vi "AlliGator Get Local Fit & Residuals.vi"(6 "Fit Options":T1={"Show Fit Residuals"=TRUE, "Fit Model"=enum."1-Exponential", "Residual Type"=enum."Standard", "Max Decay Percentile"=0.0, "Min Decay Percentile"=0.0, "Show Full Decay"=TRUE, "Weights"=enum."Unweighted", "Fitting Method"=enum."Least Square", "Compute Parameter Uncertainties"=TRUE, "Periodic Boundaries"=TRUE, "Model Calculation"=enum."Simulation", "Period"=1.2500000000000001e-08, "Termination Criteria"={"Max Iterations"=0, "Max Function Calls"=0, "Max Time"=1000.0, "Function Tolerance"=1e-06, "Parameter Tolerance"=1e-06, "Gradient Tolerance"=0.0, "Min Lambda"=1e-06, "Max Lambda"=1e-06, "Initial Tick Count"=0}, "Offset Resolution"=1.2500000000000001e-08, "Use Local IRF"=TRUE, "Fitting Algorithm"=enum."Levenberg-Marquardt"} {"Offset Resolution" min=0.0; "Period" min=0.0; "Min Decay Percentile" min=0.0 max=1.0; "Max Decay Percentile" min=0.0 max=1.0}, 7 "Use Normalized IRF (T)":bool=TRUE, 8 "Error In":errorcluster, 9 "All Fit Parameters (w tau)":dbl[](array[numeric]), 10 "IRF":cluster{"X Array":dbl[], "Y Array":dbl[]}, 11 "Decay Plot":cluster{"X Array":dbl[], "Y Array":dbl[]}) -> (0 "Error Out":errorcluster, 1 "Fit Model":T2, 2 "Residual Plot":cluster{"X Array":dbl[], "Y Array":dbl[]}, 3 "Fit Plot":cluster{"X Array":dbl[], "Y Array":dbl[]})   [LabVIEW 2021, in "AlliGator Local Decay Window.lvlib"]
doc: "Gets the fit and residuals for the selected ROI."
uses:
  AlliGator Local Decay Window.lvlib
  Fits/Decay Convolution/Decay Model.ctl
  Fits/IRF(X)PSED/Decay Fit Options v2.ctl
  Fits/Residual Type.ctl
  Fits/IRF(X)PSED/Fit Weights Type.ctl
  Fits/Non-linear Fitting Method v2.ctl
  Fits/Fit Calculation Method.ctl
  Fits/Non-linear Fitting Algorithm.ctl
  AlliGator Settings List.ctl
  Variant/Variant to Data/Variant to Boolean.vi
  AlliGator Settings.lvlib
  Fits/Fits.lvlib
  Variant/Variant to Data/Variant to Data.lvlib
  AlliGator Decay Fit.lvlib
panel:
  # "see the AlliGator License on the block diagram (Ctrl+E or Window:Show Block Diagram)"
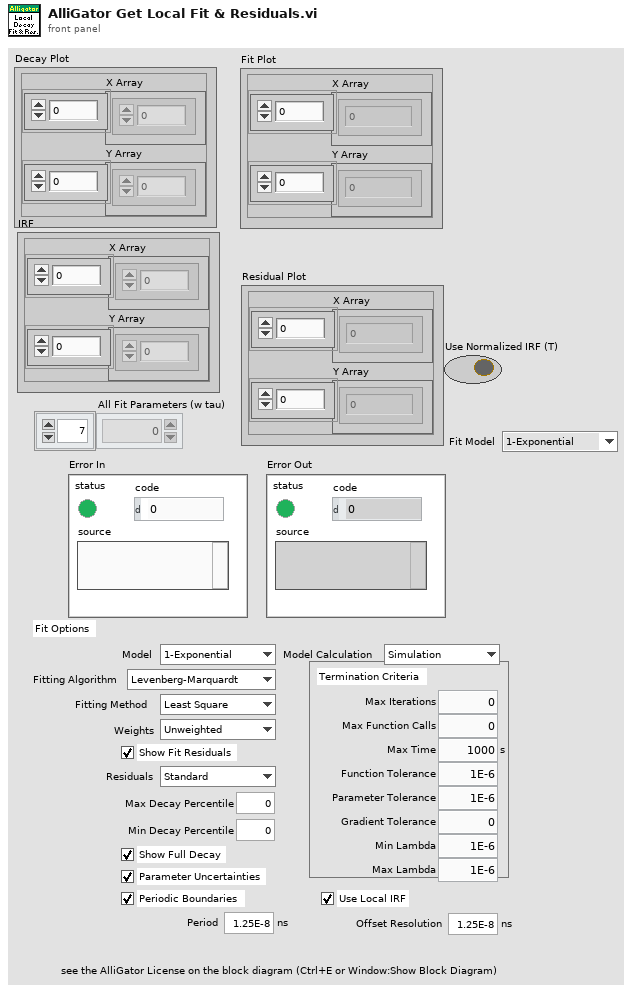
[diagram p1: front panel]
types:
  T1 = typedef "Fits.lvlib/Decay Fit Options v2.ctl" = cluster{"Show Fit Residuals":bool, "Fit Model":T2, "Residual Type":T3, "Max Decay Percentile":dbl, "Min Decay Percentile":dbl, "Show Full Decay":bool, "Weights":T4, "Fitting Method":T5, "Compute Parameter Uncertainties":bool, "Periodic Boundaries":bool, "Model Calculation":T6, "Period":dbl[unit], "Termination Criteria":cluster{"Max Iterations":i32, "Max Function Calls":i32, "Max Time":dbl[unit], "Function Tolerance":dbl, "Parameter Tolerance":dbl, "Gradient Tolerance":dbl, "Min Lambda":dbl, "Max Lambda":dbl, "Initial Tick Count":u32}, "Offset Resolution":dbl[unit], "Use Local IRF":bool, "Fitting Algorithm":T7}
  T2 = typedef "Fits.lvlib/Decay Model.ctl" = enum16{"1-Exponential", "2-Exponentials"}
  T3 = typedef "Fits.lvlib/Residual Type.ctl" = enum16{"Standard", "Normalized", "Reduced"}
  T4 = typedef "Fits.lvlib/Fit Weights Type.ctl" = enum16{"Unweighted", "1/Variance", "Best of All"}
  T5 = typedef "Fits.lvlib/Non-linear Fitting Method v2.ctl" = enum16{"Least Square", "Least Absolute Residual", "Bisquare", "MLE", "-", "Best of All"}
  T6 = typedef "Fits.lvlib/Fit Calculation Method.ctl" = enum16{"Simulation", "Convolution", "Integration"}
  T7 = typedef "Fits.lvlib/Non-linear Fitting Algorithm.ctl" = enum16{"Levenberg-Marquardt", "Trust-Region Dogleg"}
  T8 = typedef "AlliGator Settings.lvlib/AlliGator Settings List.ctl" = enum16{"GUI:Visible Settings Tab", "GUI:Last Run Version", "Source Image:Use Image Histogram for Contrast", "Source Image:Low Count Pixels Rejection Options", "Source Image:High Count Pixels Rejection Options", "Source Image:Use Image Brightness", "Source Image:Blend Overlay with Image Background", "Source Image:Use Fixed ROI Diameter", "Source Image:ROI Diameter", "Source Image:ROI Center Color", "Source Image:Peak Threshold", "Source Image:Intensity Threshold", "Source Image:Image Binning Options", "Source Image:Image Smoothing Options", "Source Image:Image Histogram Active", "Source Image:Invert Binary Mask", "Source Image:Hot Pixel Removal", "Source Image:Overlay Analyzed ROI Center", "Source Image:Auto-Adjust Contrast", "Source Image:Histogram Lower Percentile", "Source Image:Histogram Upper Percentile", "Source Image:Save Source Image", "Source Image:Scale Bar Options", "Source Image:Image Resolution (Pixel Size)", "Source Image:Flatfield Correction", "Source Image:Show Dead Left Columns Correction", "Source Image:Dead Left Columns Correction", "Source Image:Image Pre-Processing Operations Order", "Data Information:Gate Width", "Data Information:Nanotime Gate Separation", "Data Information:Macrotime Gate Separation", "Data Information:Gate Step", "Data Information:# Gates", "Data Information:Gate Image Exposure", "Data Information:Gate Image Integration", "Data Information:Gates to Skip", "Data Information:Gates to Keep", "Data Information:Define Gates to", "Data Information:Channel Name", "Data Information:Available Channel Names", "Data Information:Channel Arithmetic", "Data Information:Background File Subtraction", "Data Information:Background File", "Data Information:Background Scaling Factor", "Data Information:Background Pile-up Correction", "Data Information:Background Pixel Well Capacity", "Data Information:Laser Period", "Data Information:SYNC Period", "Data Information:Pile-up Correction", "Data Information:Pixel Well Capacity", "Data Information:Dataset Scaling Factor", "Fluorescence Decay_Decay Pre-Processing:Reverse Gates", "Fluorescence Decay_Decay Pre-Processing:Verbose Decay Pre-Processing", "Fluorescence Decay_Decay Pre-Processing:Use Decay Pre-Processing", "Fluorescence Decay_Decay Pre-Processing:Background Subtraction", "Fluorescence Decay_Decay Pre-Processing:Background Definition Range", "Fluorescence Decay_Decay Pre-Processing:Baseline Subtraction Method", "Fluorescence Decay_Decay Pre-Processing:Decay Pre-Processing Operations Order", "Fluorescence Decay_Decay Pre-Processing:Smoothing Parameter", "Fluorescence Decay_Decay Pre-Processing:Shift Decay", "Fluorescence Decay_Decay Pre-Processing:Decay Shift Parameters", "Fluorescence Decay_Decay Pre-Processing:Fold Decay", "Fluorescence Decay_Decay Pre-Processing:# Folds", "Fluorescence Decay_Decay Pre-Processing:1-Normalize Decay", "Fluorescence Decay_Decay Pre-Processing:[0-1]-Normalize Decay", "Fluorescence Decay_Decay Pre-Processing:Smoothen Decay", "Fluorescence Decay_Decay Pre-Processing:Extrapolate Decay", "Fluorescence Decay_Decay Pre-Processing:Use Periodicity", "Fluorescence Decay_Decay Pre-Processing:Use Cursors", "Fluorescence Decay_Decay Pre-Processing:Tail Fraction", "Fluorescence Decay_Decay Pre-Processing:Head Fraction", "Fluorescence Decay_Decay Pre-Processing:Additional Points", "Fluorescence Decay_Decay Pre-Processing:Straighten Decay", "Fluorescence Decay_Decay Pre-Processing:Constant Background", "Fluorescence Decay_Decay Pre-Processing:Pixel-Normalize Decay", "Fluorescence Decay_Advanced Analysis:Extract IRF instead of Decay", "Fluorescence Decay_Advanced Analysis:IRF Extraction Options", "Fluorescence Decay_Advanced Analysis:IRF Optimization Options", "Fluorescence Decay_Advanced Analysis:Square Pulse Options", "Fluorescence Decay_Advanced Analysis:IRF Order", "Fluorescence Decay_Advanced Analysis:IRF Time Constants", "Fluorescence Decay_Advanced Analysis:Wavelet Analysis Options", "Fluorescence Decay_Advanced Analysis:Average Lifetime Options", "Fluorescence Decay_Fit Options:Fit Options", "Fluorescence Decay_Fit Options:Use Legacy Fitting Approach", "Fluorescence Decay_Fit Options:Use Data Information Laser Period", "Fluorescence Decay_Fit Parameters:Displayed Fit Parameters", "Fluorescence Decay_Fit Parameters:Fit Parameter Constraints", "Fluorescence Decay_Fit Parameters:Export Tabulated Results", "Fluorescence Decay_Fit Parameters:MLE Baseline Offset Type", "Fluorescence Decay_Fit Parameters:MLE Baseline Offset", "Fluorescence Decay_Fit Parameters:Guess Parameter Names", "Fluorescence Decay_Fit Parameters:Guess Parameter Values", "Fluorescence Decay_Fit Parameters:Guess Parameters Options", "Fluorescence Decay_Styles:Show Last Decay Only", "Fluorescence Decay_Styles:Decay Graph Color Array", "Fluorescence Decay:Decay Graph Active", "Fluorescence Decay Statistics:Min Peak Value", "Fluorescence Decay Statistics:Reject Low Decay Peak Pixels", "Fluorescence Decay Statistics:Reject High Decay Peak Pixels", "Fluorescence Decay Statistics:Max Peak Value", "Time Traces:Use File Timestamp", "Time Traces:Time Step", "Time Traces:Use Intensity Correction File", "Time Traces:Intensity Correction File", "Phasor Plot:Phasor Plot Smoothing Options", "Phasor Plot:Phasor Plot Size", "Phasor Plot:Phasor Plot Graphics Options", "Phasor Plot:Cumulative Phasor Plot", "Phasor Plot:Use Phasor Brightness", "Phasor Plot:Blend Overlay with Phasor Background", "Phasor Plot:Save Phasor Plot", "Phasor Plot:Show References", "Phasor Plot:Phasor Ratio Decay Range", "Phasor Plot:Exponential Fading", "Phasor Plot:Phasor Ratio Reference Colors", "Phasor Plot:Reference Radius", "Phasor Plot:Show Color Map Vertices", "Phasor Plot:Phasor Plot Active", "Phasor Plot:Phasor Ratio Color Map Type", "Phasor Plot:Phasor Ratio Color Map", "Phasor Plot:Phasor Ratio Display Range", "Phasor Plot:Selected Image ROI(s)", "Phasor Plot:All Image ROIs", "Phasor Plot:Selected Phasor Plot ROI(s)", "Phasor Plot:All Phasor Plot ROIs", "Phasor Plot:Phasor Ratio Color-Coded Quantity", "Phasor Plot:Store Phasor Harmonics", "Phasor Plot:Draw Reference Segment", "Phasor Plot:User-Defined Quantity", "Phasor Graph:Phasor Frequency", "Phasor Graph:Phasor Ratio Type", "Phasor Graph:Pixel-level Phasor Computation", "Phasor Graph:Save Phasor Graph", "Phasor Graph:Phasor Graph Active", "Phasor Graph:Phasor SDV Options", "Phasor Calibration:Use Backup Calibration if needed", "Phasor Graph:Define Shortest Lifetime as", "Phasor Calibration:Backup Calibration Type", "Phasor Calibration:Calibration Type", "Phasor Calibration:Calibration Lifetime", "Phasor Calibration:Calibration Map Algorithm", "Single-Exponential Phasor Locus (SEPL):Gate Parameters", "Single-Exponential Phasor Locus (SEPL):User-defined Gate", "Single-Exponential Phasor Locus (SEPL):User-defined IRF", "Single-Exponential Phasor Locus (SEPL):Phasor Parameters", "Single-Exponential Phasor Locus (SEPL):Decay & IRF Parameters", "Single-Exponential Phasor Locus (SEPL):Display Parameters", "Lifetime Analysis:Decay Analysis Parameters", "Lifetime Analysis:Lifetime Map Active", "Plugins:Python Settings", "Miscellaneous:Verbose Mode", "Miscellaneous:Beep after Script", "Miscellaneous:Saved Image File Format", "Miscellaneous:Exported Gate Image Settings", "Miscellaneous:Include Loading in Timing", "Miscellaneous:Verbose Settings Mode", "Miscellaneous:Histogram Options", "Miscellaneous:Beep on Error", "Miscellaneous:# Logical Processors Used", "Miscellaneous:ROI Description Max Characters", "Miscellaneous:Verbose Error Mode", "Miscellaneous:Transparent Mask Color"}
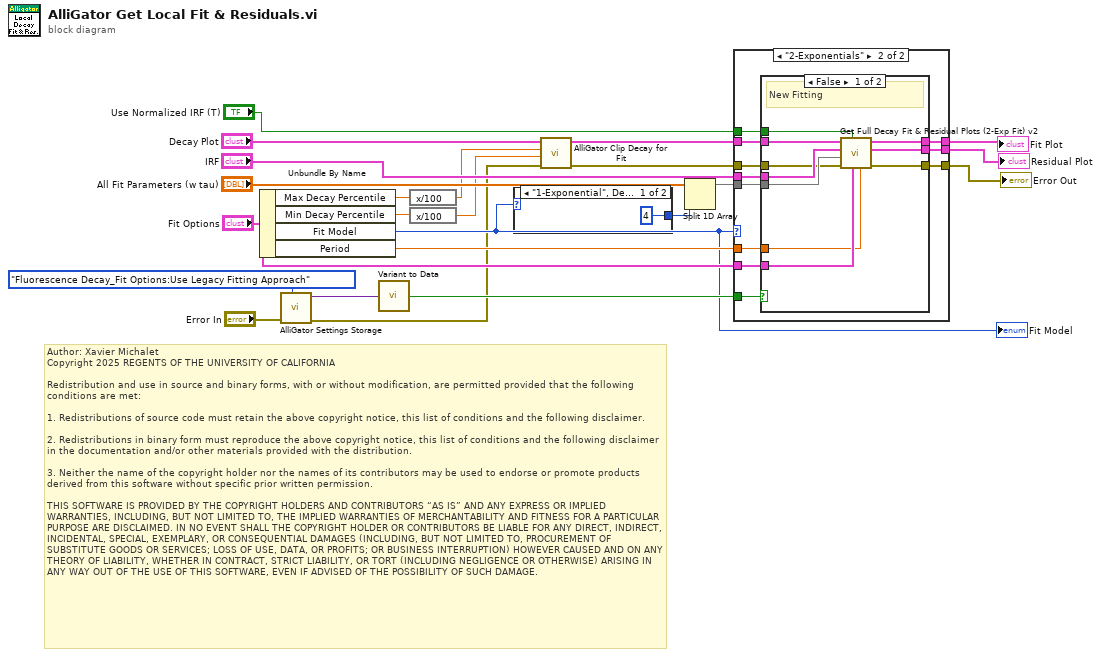
[diagram p0: block diagram]
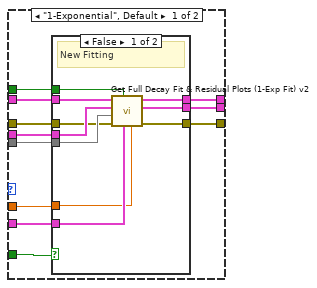
[diagram p2: hidden frame]
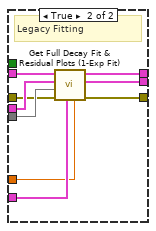
[diagram p3: hidden frame]
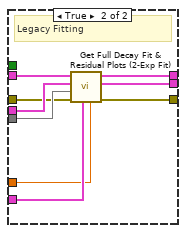
[diagram p4: hidden frame]
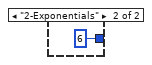
[diagram p5: hidden frame]
diagram:
  # "Author: Xavier Michalet\nCopyright 2025 REGENTS OF THE UNIVERSITY OF CALIFORNIA\n\nRedistribution and use in source and binary forms, with or without modification, are permitted provided that the following conditions are met:\n\n1. Redistributions of source code must retain the above copyright notice, this list of conditions and the following disclaimer.\n\n2. Redistributions in binary form must reproduce the above copyright notice, this list of conditions and the following disclaimer in the documentation and/or other materials provided with the distribution.\n\n3. Neither the name of the copyright holder nor the names of its contributors may be used to endorse or promote products derived from this software without specific prior written permission.\n\nTHIS SOFTWARE IS PROVIDED BY THE COPYRIGHT HOLDERS AND CONTRIBUTORS “AS IS” AND ANY EXPRESS OR IMPLIED WARRANTIES, INCLUDING, BUT NOT LIMITED TO, THE IMPLIED WARRANTIES OF MERCHANTABILITY AND FITNESS FOR A PARTICULAR PURPOSE ARE DISCLAIMED. IN NO EVENT SHALL THE COPYRIGHT HOLDER OR CONTRIBUTORS BE LIABLE FOR ANY DIRECT, INDIRECT, INCIDENTAL, SPECIAL, EXEMPLARY, OR CONSEQUENTIAL DAMAGES (INCLUDING, BUT NOT LIMITED TO, PROCUREMENT OF SUBSTITUTE GOODS OR SERVICES; LOSS OF USE, DATA, OR PROFITS; OR BUSINESS INTERRUPTION) HOWEVER CAUSED AND ON ANY THEORY OF LIABILITY, WHETHER IN CONTRACT, STRICT LIABILITY, OR TORT (INCLUDING NEGLIGENCE OR OTHERWISE) ARISING IN ANY WAY OUT OF THE USE OF THIS SOFTWARE, EVEN IF ADVISED OF THE POSSIBILITY OF SUCH DAMAGE."
  n1 = Unbundle By Name("Fit Options") -> ("Max Decay Percentile"=w8:dbl, "Min Decay Percentile"=w3:dbl, "Fit Model"=w12:T2, "Period"=w19:dbl[unit])
  "Fit Model" <- w12
  n2 = call "AlliGator Settings Storage.vi"("AlliGator Settings List"=AlliGator_Settings_List."Fluorescence Decay_Fit Options:Use Legacy Fitting Approach", "Error In"="Error In") -> ("Error Out"=w7:errorcluster, "Variant Data out"=w16:variant)  [unwired: 8 in]
  n3 = call-poly "Variant to Data.vi"("Variant"=w16) -> ("Value"=w15:bool)  [unwired: 8 in]
  n4 = expression code="x/100"(w8) -> (w4:dbl)
  n5 = expression code="x/100"(w3) -> (w2:dbl)
  n6 = case shown="\"1-Exponential\", Default" w12 {
    tunnel: [4 ("index") 6 ("index")] -> w11
    frame "1-Exponential", Default {
    }
    frame "2-Exponentials" {
    }
  }
  n7 = call "AlliGator Clip Decay for Fit.vi"("Error In"=w7, "Min Decay Percentile (0)"=w2, "Max Decay Percentile (1)"=w4, "Decay in"="Decay Plot") -> ("Error Out"=w5:errorcluster, "Clipped Decay out"=w6:cluster{"t Array":dbl[], "Value Array":dbl[]})  [unwired: 3 in, 3 out]
  n8 = Split 1D Array(array="All Fit Parameters (w tau)", index=w11) -> (first subarray=w10:dbl[])  [unwired: 1 out]
  n9 = case shown="\"2-Exponentials\"" w12 {
    tunnel: w6 -> [w36 w66]
    tunnel: "IRF" -> [w35 w65]
    tunnel: w10 -> [w34 w64]
    tunnel: "Fit Options" -> [w30 w63]
    tunnel: [w32 w62] -> w22
    tunnel: [w31 w61] -> w21
    tunnel: [w33 w60] -> w20
    tunnel: w19 -> [w29 w59]
    tunnel: w15 -> [w28 w58]
    tunnel: w5 -> [w27 w57]
    tunnel: "Use Normalized IRF (T)" -> [w26 w56]
    frame "1-Exponential", Default {
      n10 = case shown="False" w28 {
        tunnel: w36 -> [w46 w55]
        tunnel: w35 -> [w45 w54]
        tunnel: w34 -> [w44 w53]
        tunnel: w27 -> [w43 w52]
        tunnel: [w38 w51] -> w33
        tunnel: [w40 w50] -> w32
        tunnel: [w39 w49] -> w31
        tunnel: w30 -> [w42 w48]
        tunnel: w29 -> [w41 w47]
        tunnel: w26 -> [w37 _]
        frame False {
          # "New Fitting"
          n11 = call "Get Full Decay Fit & Residual Plots (1-Exp Fit) v2.vi"("SYNC Period"=w41, "Fit Options"=w42, "Use Normalized IRF (T)"=w37, "Error In"=w43, "Best Fit Parameters (w tau)"=w44, "IRF"=w45, "Full Decay"=w46) -> ("Error Out"=w38:errorcluster, "Full Decay Residuals"=w39:cluster{"t Array":dbl[], "Y Array":dbl[]}, "Full Fitted Decay"=w40:cluster{"t Array":dbl[], "Y Array":dbl[]})  [unwired: 2 in]
        }
        frame True {
          # "Legacy Fitting"
          n12 = call "Get Full Decay Fit & Residual Plots (1-Exp Fit).vi"("Laser Period"=w47, "Fit Options"=w48, "Error In"=w52, "Best Fit Parameters (All)"=w53, "IRF"=w54, "Full Decay"=w55) -> ("Error Out"=w51:errorcluster, "Full Decay Residuals"=w49:cluster{"t Array":dbl[], "Y Array":dbl[]}, "Full Fitted Decay"=w50:cluster{"t Array":dbl[], "Y Array":dbl[]})  [unwired: 3 in]
        }
      }
    }
    frame "2-Exponentials" {
      n13 = case shown="False" w58 {
        tunnel: w66 -> [w76 w85]
        tunnel: w65 -> [w75 w84]
        tunnel: w64 -> [w74 w83]
        tunnel: w63 -> [w73 w82]
        tunnel: [w70 w81] -> w62
        tunnel: [w71 w80] -> w61
        tunnel: [w72 w79] -> w60
        tunnel: w59 -> [w69 w78]
        tunnel: w57 -> [w68 w77]
        tunnel: w56 -> [w67 _]
        frame False {
          # "New Fitting"
          n14 = call "Get Full Decay Fit & Residual Plots (2-Exp Fit) v2.vi"("SYNC Period"=w69, "Fit Options"=w73, "Use Normalized IRF (T)"=w67, "Error In"=w68, "Best Fit Parameters (w tau)"=w74, "IRF"=w75, "Full Decay"=w76) -> ("Error Out"=w72:errorcluster, "Full Decay Residuals"=w71:cluster{"t Array":dbl[], "IRF Array":dbl[]}, "Full Fitted Decay"=w70:cluster{"t Array":dbl[], "IRF Array":dbl[]})  [unwired: 2 in]
        }
        frame True {
          # "Legacy Fitting"
          n15 = call "Get Full Decay Fit & Residual Plots (2-Exp Fit).vi"("Laser Period"=w78, "Fit Options"=w82, "Error In"=w77, "Best Fit Parameters"=w83, "IRF"=w84, "Full Decay"=w85) -> ("Error Out"=w79:errorcluster, "Full Decay Residuals"=w80:cluster{"t Array":dbl[], "IRF Array":dbl[]}, "Full Fitted Decay"=w81:cluster{"t Array":dbl[], "IRF Array":dbl[]})  [unwired: 3 in]
        }
      }
    }
  }
  "Error Out" <- w20
  "Fit Plot" <- w22
  "Residual Plot" <- w21
